vi "eFGV - Template.vi"(6 "State - eFGV":T1=enum."Close", 8 "error in (no error)":errorcluster) -> (0 "error out":errorcluster)   [LabVIEW 2020]
uses:
  Control/State - eFGV.ctl
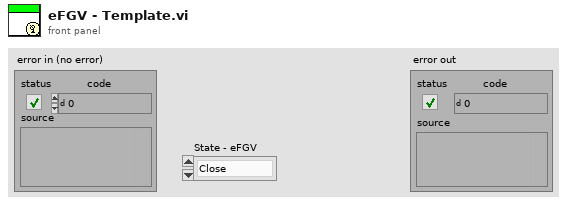
[diagram p1: front panel]
types:
  T1 = typedef "State - eFGV.ctl" = enum16{"Init", "Read", "Write", "Close"}
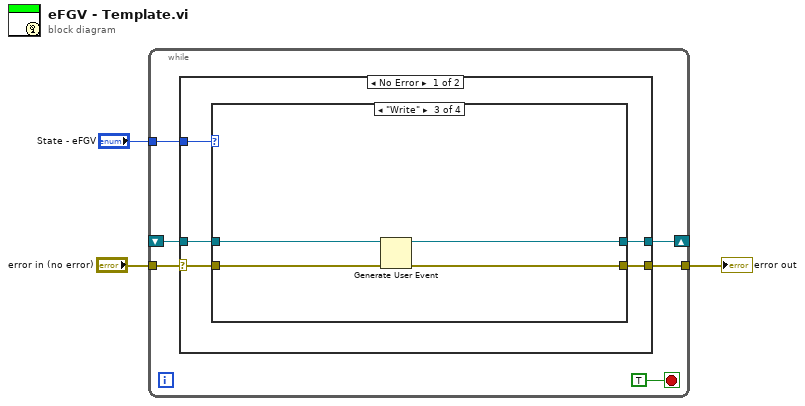
[diagram p0: block diagram]
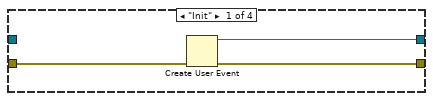
[diagram p2: hidden frame]
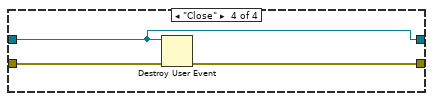
[diagram p4: hidden frame]
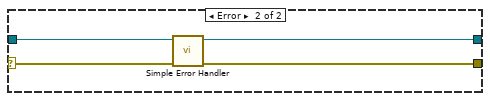
[diagram p5: hidden frame]
diagram:
  n1 = while {
    tunnel: "State - eFGV" -> [w8]
    tunnel: "error in (no error)" -> [w7]
    tunnel: [w6] -> w1
    shift-right: [w5] -> _
    shift-left: _ -> [w4]
    stop <- TRUE stop-if-true
    n2 = case shown="No Error" w7 {
      selector: w7 -> [w13 w29]
      tunnel: w8 -> [w14 _]
      tunnel: [w12 w27] -> w6
      tunnel: [w11 w28] -> w5
      tunnel: w4 -> [w10 w28]
      frame No Error {
        n3 = case shown="\"Write\"" w14 {
          tunnel: w13 -> [w17 w19 w23 w26]
          tunnel: [w16 w19 w22 w25] -> w12
          tunnel: [w15 w18 w21 w24] -> w11
          tunnel: w10 -> [_ w18 w20 w24]
          frame "Init" {
            n4 = Create User Event(error in=w17) -> (user event=w15:refnum<user-event>, error out=w16:errorcluster)  [unwired: 1 in]
          }
          frame "Read", Default {
          }
          frame "Write" {
            n5 = Generate User Event(user event=w20, error in=w23) -> (user event out=w21:refnum<user-event>, error out=w22:errorcluster)  [unwired: 2 in]
          }
          frame "Close" {
            n6 = Destroy User Event(user event=w24, error in=w26) -> (error out=w25:errorcluster)
          }
        }
      }
      frame Error {
        n7 = call <vilib>:"Simple Error Handler.vi"("error in (no error)"=w29) -> ("error out"=w27:errorcluster)  [unwired: 4 in, 4 out]
      }
    }
  }
  "error out" <- w1
